vi "getTestsFromTestCaseByClassPath.vi"(8 "error in":errorcluster, 10 "TestCase Path":path) -> (0 "error out":errorcluster, 1 "test paths":path[](array[path]), 2 "tests":string[](array[string]))   [LabVIEW 2013, in "TestLoader.lvclass"]
uses:
  TestLoader.lvclass
  Libraries/VITesterUtilities.lvlib
panel:
  # "JKI VI Tester for LabVIEW\nhttp://jkisoft.com/vi-tester\nCopyright (C) 2007-2009, JKI <info@jkisoft.com>\nALL RIGHTS RESERVED"
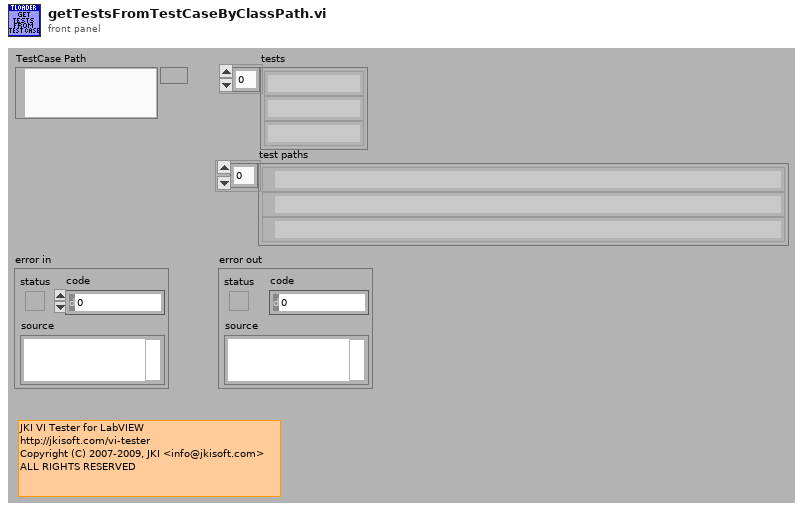
[diagram p1: front panel]
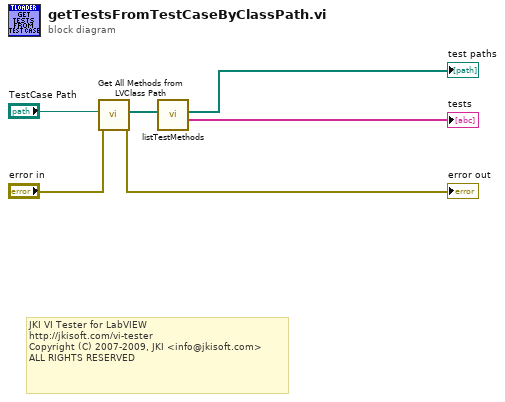
[diagram p0: block diagram]
diagram:
  # "JKI VI Tester for LabVIEW\nhttp://jkisoft.com/vi-tester\nCopyright (C) 2007-2009, JKI <info@jkisoft.com>\nALL RIGHTS RESERVED"
  n1 = call "Get All Methods from LVClass Path.vi"("error in"="error in", "class path"="TestCase Path") -> ("error out"=→"error out":errorcluster, "Methods"=w4:path[])  [unwired: 8 in]
  n2 = call "listTestMethods.vi"("Methods"=w4) -> ("Test Method Names"=→"tests":string[], "Test Method Paths"=→"test paths":path[])  [unwired: 9 in]
